vi "brace_space_inside_brace_solution.vi"(8 "error in (no error)":errorcluster, 11 "Instrument Command In":string=" :TRIGger:AND:ENABle {{ON | 1} | {OFF | 0}}") -> (0 "error out":errorcluster, 3 "Instrument Command Out":string)   [LabVIEW 2018]
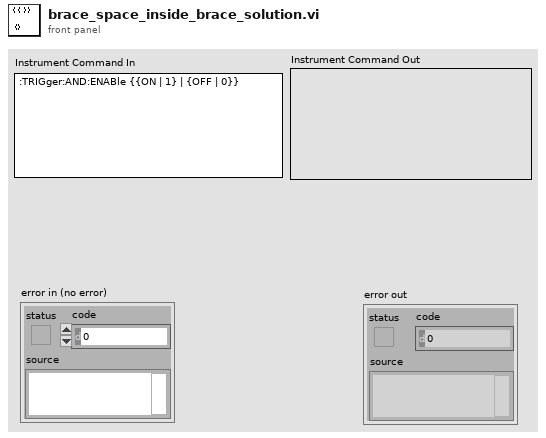
[diagram p1: front panel]
types:
  T1 = cluster{"Start Sting":string, "End String":string}[]
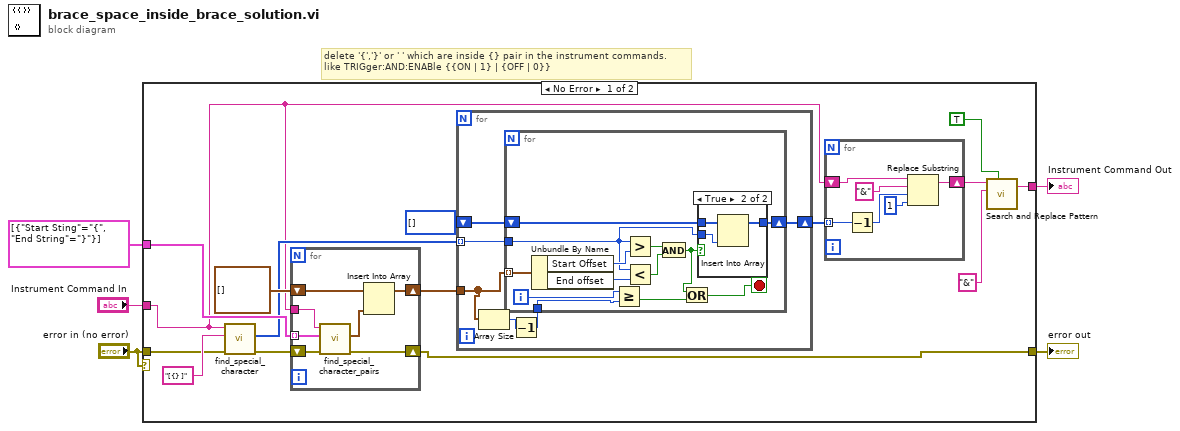
[diagram p0: block diagram]
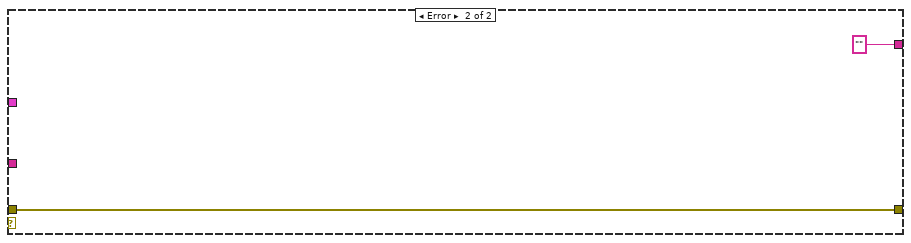
[diagram p3: hidden frame]
diagram:
  # "delete '{','}' or ' ' which are inside {} pair in the instrument commands.\nlike TRIGger:AND:ENABle {{ON | 1} | {OFF | 0}}"
  n1 = case shown="No Error" "error in (no error)" {
    tunnel: T1 [{"Start Sting"="{", "End String"="}"}] -> [w19 _]
    tunnel: "Instrument Command In" -> [w7 _]
    tunnel: [w8 "" ("result string")] -> w3
    tunnel: "error in (no error)" -> [w6 w58]
    tunnel: [w9 w58] -> w2
    frame No Error {
      n2 = call "find_special_character.vi"("error in (no error)"=w6, "Character"="[{} ]" ("Start Character"), "Command String"=w7) -> ("error out"=w10:errorcluster, "Offset Array"=w17:i32[])  [unwired: 7 out]
      n3 = for {
        tunnel: w7 -> [w56]
        tunnel: w19 -> [w55] mode=indexing
        shift-right: [w52] -> w16
        shift-left: cluster{"Start Offset":i32, "End offset":i32}[] [] ("Pair Offset") -> [w53]
        shift-right: [w50] -> w9
        shift-left: w10 -> [w51]
        n4 = call "find_special_character_pairs.vi"("error in (no error)"=w51, "String Pair"=w55, "Command String"=w56) -> ("error out"=w50:errorcluster, "Pair Offset"=w54:cluster{"Start Offset":i32, "End offset":i32}[])  [unwired: 7 out]
        n5 = Insert Into Array(array=w53, new element=w54) -> (w52:cluster{"Start Offset":i32, "End offset":i32}[])  [unwired: 1 in]
      }
      n6 = for {
        tunnel: w17 -> [w32] mode=indexing
        tunnel: w16 -> [w29]
        shift-right: [w30] -> w14
        shift-left: i32[] [] -> [w31]
        n7 = Array Size(array=w29) -> (size(s)=w28:i32)
        n8 = Decrement(x=w28) -> (x-1=w27:i32)
        n9 = for {
          tunnel: w32 -> [w39]
          tunnel: w29 -> [w45] mode=indexing
          shift-right: [w38] -> w30
          shift-left: w31 -> [w40]
          tunnel: w27 -> [w36]
          i -> [w37]
          stop <- w33 stop-if-true
          n10 = Unbundle By Name(w45) -> ("Start Offset"=w44:i32, "End offset"=w43:i32)
          n11 = Greater Or Equal?(x=w37, y=w36) -> (x >= y?=w34:bool)
          n12 = Greater?(x=w39, y=w44) -> (0:w42:bool)
          n13 = Less?(x=w39, y=w43) -> (x < y?=w41:bool)
          n14 = And(x=w42, y=w41) -> (x .and. y?=w35:bool)
          n15 = Or(x=w35, y=w34) -> (x .or. y?=w33:bool)
          n16 = case shown="True" w35 {
            tunnel: w40 -> [w46 w49]
            tunnel: w39 -> [_ w48]
            tunnel: [w46 w47] -> w38
            frame False {
            }
            frame True {
              n17 = Insert Into Array(array=w49, new element=w48) -> (w47:i32[])  [unwired: 1 in]
            }
          }
        }
      }
      n18 = for {
        tunnel: w14 -> [w25] mode=indexing
        shift-right: [w22] -> w13
        shift-left: w7 -> [w26]
        n19 = Decrement(x=w25) -> (x-1=w21:i32)
        n20 = Replace Substring(2:1 ("length (len. of substring)"), 3:w21, 4:"&" ("substring (\"\")"), 5:w26) -> (1:w22:string)  [unwired: 1 out]
      }
      n21 = call <vilib>:"Search and Replace Pattern.vi"("string"=w13, "regular expression (\"\")"="&" ("regular expression (\"\")"), "replace all? (F)"=TRUE) -> ("result string"=w8:string)  [unwired: 1 in, 2 out]
    }
    frame Error {
    }
  }
  "Instrument Command Out" <- w3
  "error out" <- w2
